vi "Get SMO Name.vi"(8 "error in (no error)":errorcluster, 11 "Instrument.Aerotech":refnum<class "Instrument.Aerotech.lvclass">) -> (0 "error out":errorcluster, 2 "SMO Name":string, 3 "Instrument.Aerotech out":refnum<class "Instrument.Aerotech.lvclass">)   [LabVIEW 2019, in "Instrument.Aerotech.lvclass"]
uses:
  Instrument.Aerotech.lvclass
  <userlib>/LevyLab/Instrument Framework/Instrument Types/Delay Line/Instrument.DelayLine.lvclass
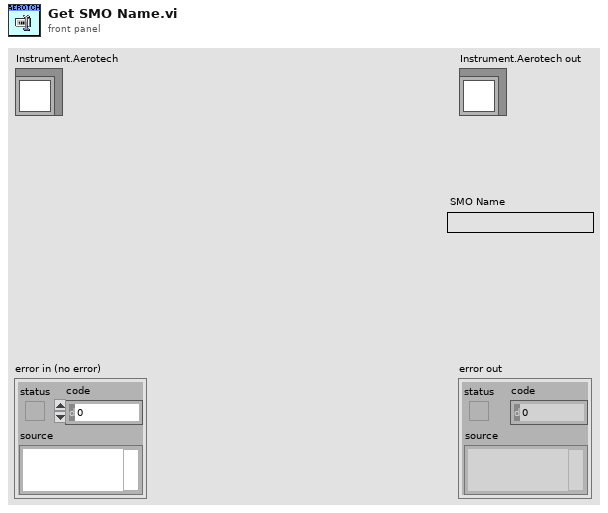
[diagram p1: front panel]
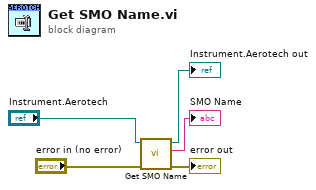
[diagram p0: block diagram]
diagram:
  n1 = call-parent "Get SMO Name.vi"("error in (no error)"="error in (no error)", "Instrument in"="Instrument.Aerotech") -> ("error out"=→"error out":errorcluster, "SMO Name"=→"SMO Name":string, "Instrument out"=→"Instrument.Aerotech out":refnum<class "Instrument.Aerotech.lvclass">)  [unwired: 7 in]
